vi "Write CurrentCommand.vi"(8 "error in (no error)":errorcluster, 10 "Command.lvclass":refnum<class "Command.lvclass">, 11 "System in":refnum<class "System.lvclass">) -> (0 "error out":errorcluster, 3 "System out":refnum<class "System.lvclass">)   [LabVIEW 2013, in "System.lvclass"]
uses:
  System.lvclass
  Commands/Command/Command.lvclass
  System.lvclass/System.ctl
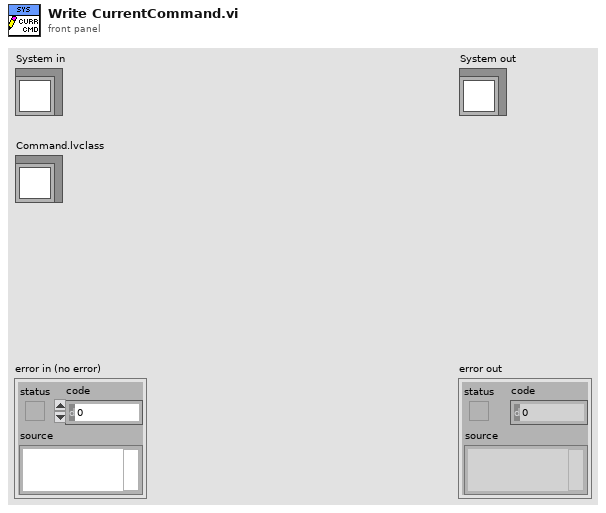
[diagram p1: front panel]
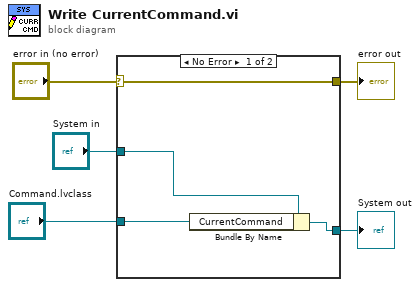
[diagram p0: block diagram]
diagram:
  n1 = case shown="No Error" "error in (no error)" {
    selector: "error in (no error)" -> [w6 w10]
    tunnel: [w6 w10] -> w4
    tunnel: [w9 w11] -> w2
    tunnel: "System in" -> [w8 w11]
    tunnel: "Command.lvclass" -> [w7 _]
    frame No Error {
      n2 = Bundle By Name(cluster=w8, "CurrentCommand"=w7) -> (w9:refnum<class "System.lvclass">)
    }
    frame Error {
    }
  }
  "error out" <- w4
  "System out" <- w2
